vi "Filter.vi"(0 "Array":cdb[](array[numeric]), 5 "Numeric":i32) -> (4 "mean":cdb[](array[numeric]))   [LabVIEW 2025]
uses:
  <vilib>/Analysis/1siggen.llb/Ramp Pattern by Samples.vi
  <vilib>/Analysis/NI_AALBase.lvlib
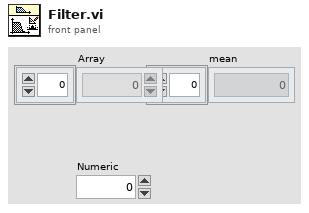
[diagram p1: front panel]
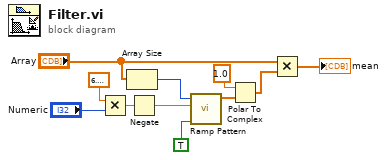
[diagram p0: block diagram]
diagram:
  n1 = Multiply(x=6.283185307179586, y="Numeric") -> (x*y=w3:dbl)
  n2 = Array Size(array="Array") -> (size(s)=w1:i32)
  n3 = Negate(x=w3) -> (-x=w8:dbl)
  n4 = call-poly <vilib>:"Ramp Pattern.vi"("exclude end?"=TRUE, "end"=w8, "samples"=w1) -> ("Ramp Pattern"=w6:dbl[])  [unwired: 7 in, 1 out]
  n5 = Polar To Complex(1:w6, 2:1.0 ("cycles")) -> (0:w7:cdb[])
  n6 = Multiply(x="Array", y=w7) -> (x*y=→"mean":cdb[])
